vi "Demo.vi"() -> ()   [LabVIEW 2016]
uses:
  Shakespear Monkeys/Gene/Character.lvclass
  C:/Users/J51654/My Projects/Evolutionary Programming/GA Framework/IGene/IGene.lvclass
  Shakespear Monkeys/Chromosome/Sentence.lvclass
  C:/Users/J51654/My Projects/Evolutionary Programming/GA Framework/IChromosome/IChromosome.lvclass
  IPopulation/IPopulation.lvclass
  IPopulation/IPopulation.lvclass/IPopulation.ctl
  IChromosome/IChromosome.lvclass/IChromosome.ctl
  Shakespear Monkeys/Gene/Character.lvclass/Character.ctl
  IChromosome/IChromosome.lvclass
  IGene/IGene.lvclass
panel:
  out "Best Fit":string
  out "X-Somes":string[](array[string])
  out "Generations":i32
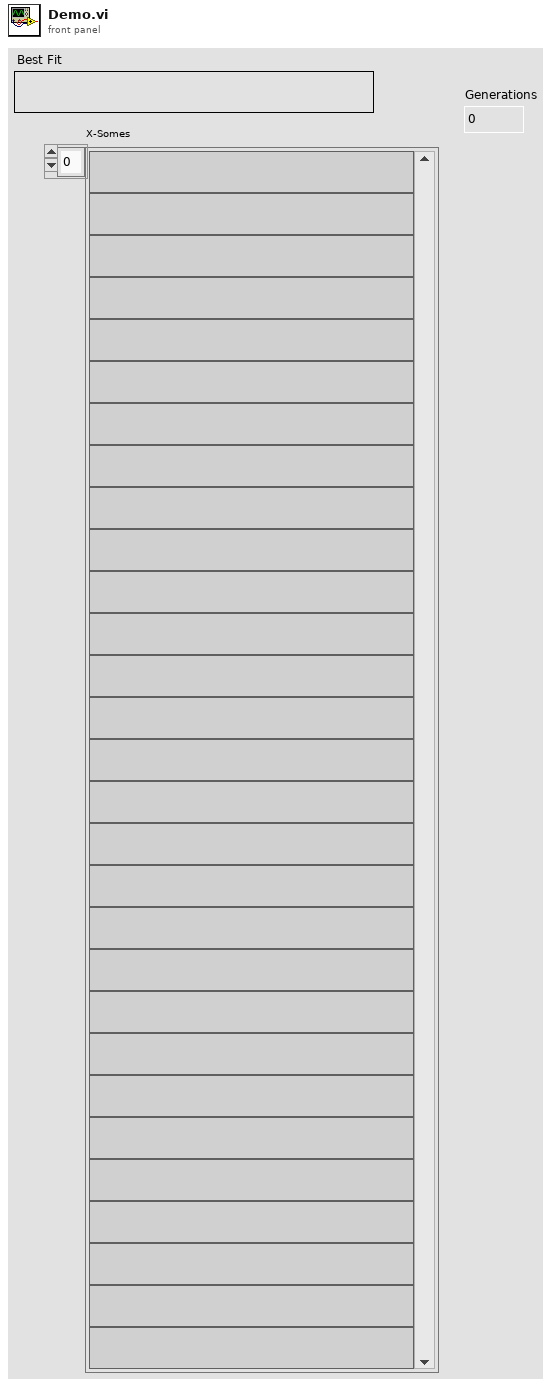
[diagram p1: front panel]
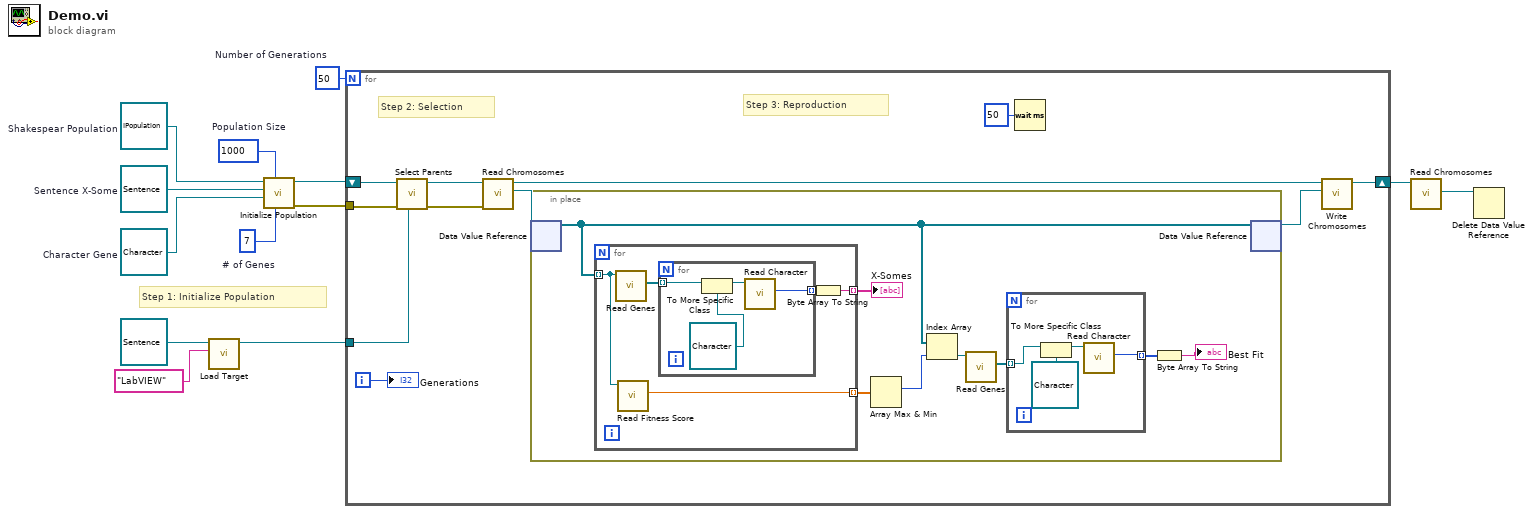
[diagram p0: block diagram]
diagram:
  w4 = 50  # Number of Generations
  w9 = u32 7  # # of Genes
  w10 = u32 1000  # Population Size
  w13 = refnum<class "IPopulation.lvclass"> refnum  # Shakespear Population
  w12 = refnum<class "Sentence.lvclass"> refnum  # Sentence X-Some
  w11 = refnum<class "Character.lvclass"> refnum  # Character Gene
  # "Step 1: Initialize Population"
  n1 = call "Load Target.vi"("Target String"="LabVIEW", "Sentence in"=refnum<class "Sentence.lvclass"> refnum) -> ("Sentence out"=w6:refnum<class "Sentence.lvclass">)  [unwired: 8 in, 1 out]
  n2 = call "Initialize Population.vi"("# of Genes"=w9, "Population Size"=w10, "Gene Type"=w11, "Chromosome Type"=w12, "IPopulation in"=w13) -> ("error out"=w5:errorcluster, "IPopulation out"=w3:refnum<class "IPopulation.lvclass">)  [unwired: 5 in]
  n3 = for {
    N: w4 -> [_]
    tunnel: w6 -> [w22]
    tunnel: w5 -> [w23]
    shift-right: [w17] -> w2
    shift-left: w3 -> [w24]
    i -> [w21]
    # "Step 3: Reproduction"
    # "Step 2: Selection"
    n4 = call "Select Parents.vi"("Target Chromosome"=w22, "error in"=w23, "IPopulation in"=w24) -> ("error out"=w14:errorcluster, "IPopulation out"=w20:refnum<class "IPopulation.lvclass">)  [unwired: 7 in]
    n5 = call "Read Chromosomes.vi"("error in (no error)"=w14, "IPopulation in"=w20) -> ("Chromosomes"=w19:refnum<data-value>, "IPopulation out"=w18:refnum<class "IPopulation.lvclass">)  [unwired: 7 in, 1 out]
    n6 = in-place {
      n7 = in-place-dvr #1(w19) -> (w30:refnum<class "IChromosome.lvclass">[])  [unwired: 1 out]
      n8 = for {
        tunnel: w30 -> [w38] mode=indexing
        tunnel: [w39] -> w32 mode=indexing
        tunnel: [w37] -> w31 mode=indexing
        n9 = call "Read Genes.vi"("IChromosome in"=w38) -> ("Genes"=w41:refnum<class "IGene.lvclass">[])  [unwired: 8 in, 2 out]
        n10 = call "Read Fitness Score.vi"("IChromosome in"=w38) -> ("Fitness Score"=w37:dbl)  [unwired: 8 in, 2 out]
        n11 = for {
          tunnel: w41 -> [w45] mode=indexing
          tunnel: [w42] -> w40 mode=indexing
          n12 = To More Specific Class(target class=refnum<class "Character.lvclass"> refnum ("Character.lvclass"), reference=w45) -> (specific class reference=w43:refnum<class "Character.lvclass">)  [unwired: 1 in, 1 out]
          n13 = call "Read Character.vi"("Character in"=w43) -> ("Character"=w42:u8)  [unwired: 8 in, 2 out]
        }
        n14 = Byte Array To String(unsigned byte array=w40) -> (string=w39:string)
      }
      "X-Somes" <- w32
      n15 = Array Max & Min(array=w31) -> (max index (indices)=w29:i32)  [unwired: 3 out]
      n16 = Index Array(array=w30, index=w29) -> (element=w28:refnum<class "IChromosome.lvclass">)
      n17 = call "Read Genes.vi"("IChromosome in"=w28) -> ("Genes"=w27:refnum<class "IGene.lvclass">[])  [unwired: 8 in, 2 out]
      n18 = for {
        tunnel: w27 -> [w34] mode=indexing
        tunnel: [w33] -> w26 mode=indexing
        n19 = To More Specific Class(target class=refnum<class "Character.lvclass"> refnum ("Character.lvclass"), reference=w34) -> (specific class reference=w35:refnum<class "Character.lvclass">)  [unwired: 1 in, 1 out]
        n20 = call "Read Character.vi"("Character in"=w35) -> ("Character"=w33:u8)  [unwired: 8 in, 2 out]
      }
      n21 = Byte Array To String(unsigned byte array=w26) -> (string=→"Best Fit":string)
      n22 = in-place-dvr #1(w30) -> (w16:refnum<data-value>)  [unwired: 1 out]
    }
    n23 = Wait (ms)(milliseconds to wait=u32 50) -> ()  [unwired: 1 out]
    n24 = call "Write Chromosomes.vi"("Chromosomes"=w16, "IPopulation in"=w18) -> ("IPopulation out"=w17:refnum<class "IPopulation.lvclass">)  [unwired: 8 in, 1 out]
    "Generations" <- w21
  }
  n25 = call "Read Chromosomes.vi"("IPopulation in"=w2) -> ("Chromosomes"=w1:refnum<data-value>)  [unwired: 8 in, 2 out]
  n26 = Delete Data Value Reference(data value reference=w1) -> ()  [unwired: 1 in, 2 out]
